vi "Main Tclk.vi"() -> ()   [LabVIEW 2018] (continued)
                n4379 = local write "Faraday Cup before mill"(w3310) -> ()
                n4380 = call <vilib>:"Three Button Dialog.vi"("Allow user to close window? (TRUE)"=FALSE, "Center Button Text (\"No\")"="Manual Re-engage" ("T button name (\"OK\")"), "Left Button Text (\"Yes\")"="Auto Re-engage" ("T button name (\"OK\")"), "message"="Reheat finish and ready to re-engage?") -> ("Which Button?"=w3313:T78)  [unwired: 7 in]
                n4381 = case shown="\"Left Button\"" w3313 {
                  frame "Left Button" {
                    n4382 = stacked-sequence {
                      frame #0 {
                        w3352 = dbl[] [] ("Re-engage Delta X array")
                        w3341 = u8 0 ("Re-engage X shift")
                        w3344 = TRUE ("Auto re-engage")
                        n4383 = local read "X shift from last"() -> (w3346:dbl)
                        n4384 = local read "Y shift from last"() -> (w3350:dbl)
                        n4385 = local read "Reheat from last"() -> (w3347:bool)
                        n4386 = local read "FIB-SEM Angle"() -> (w3355:dbl)
                        n4387 = Get Date/Time In Seconds() -> (seconds since 1Jan1904=w3353:timestamp)
                        "Re-engage time" <- w3353
                        n4388 = local read "Pre-reheat time"() -> (w3356:timestamp)
                        n4389 = Subtract(x=w3353, y=w3356) -> (x-y=w3357:dbl)
                        n4390 = expression code="x/60"(w3357) -> (w3358:dbl)
                        n4391 = expression code="cos(x*pi/180)"(w3355) -> (w3354:dbl)
                        n4392 = Select(t=w3346, s=w3347, f=0.0 ("Re-engage X shift")) -> (s? t:f=w3349:dbl)
                        n4393 = Natural Logarithm(1:w3358) -> (0:w3360:dbl)
                        n4394 = local write "Status message"("Auto re-engaging ..." ("Status message")) -> ()
                        n4395 = shared-variable ".\\Zeiss Library.lvlib\\FIB PID reset"(w3344) -> ()  [unwired: 1 in, 1 out]
                        n4396 = local write "Re-engage X shift (um)"(w3349) -> ()
                        n4397 = Compound Arithmetic op=MULTIPLY(w3354, w3360, 2.5 ("value"), 0.0 ("value")) -> (w3351:dbl)
                        n4398 = Select(t=w3350, s=w3347, f=w3351) -> (s? t:f=w3345:dbl)
                        n4399 = local write "Re-engage Y shift (um)"(w3345) -> ()
                        n4400 = local read "Last milling snapshot"() -> (w3337:path)
                        n4401 = local write "Status Tabs"(T11."Status" ("Status Tabs")) -> ()
                        n4402 = call-poly <vilib>:"Read From XML File.vi"("XML File Path"=w3337) -> ("XML Elements"=w3338:string)  [unwired: 8 in, 2 out]
                        n4403 = local write "Re-engage counts"(w3341) -> ()
                        n4404 = local write "Recovered counts"(w3341) -> ()
                        n4405 = local write "Last re-engage count"(w3341) -> ()
                        n4406 = Unflatten From XML(xml string=w3338, type=T46 {"Timestamp"=timestamp(0 s since 1904-01-01), "Milling Z voltage"=0.0, "FIB slice #"=0, "Pause for reheat"=FALSE, "Last good FI"=0.0, "Focus index"=0.0, "SEM max FOV"=0.0, "Remaining X shift frames"=0, "Remaining Y shift frames"=0} ("output cluster")) -> (value=w3336:T46)  [unwired: 1 in, 1 out]
                        n4407 = local write "Image Tabs"(T37."Logging: Realtime Graphs" ("Image Tabs")) -> ()
                        n4408 = Unbundle By Name(w3336) -> ("Milling Z voltage"=w3335:sgl)
                        n4409 = shared-variable ".\\Zeiss Library.lvlib\\Milling Z Voltage Last"(w3335) -> ()  [unwired: 1 in, 1 out]
                        "Auto re-engage" <- w3344
                        "Re-engage Delta X array" <- w3352
                        "Re-engage Delta Y array" <- w3352
                        "Re-engage Y shift array" <- w3352
                        "Re-engage X shift array" <- w3352
                      }
                      frame #1 {
                        w3364 = TRUE ("Reset WD")
                        w3365 = FALSE ("Reheat")
                        n4410 = local write "Config Tabs"(T24."SEM" ("Config Tabs")) -> ()
                        n4411 = local write "Image Tabs"(T37."Detector A" ("Image Tabs")) -> ()
                        n4412 = local write "Pause for reheat"(w3365) -> ()
                        n4413 = local write "Mill Manual Pause"(w3365) -> ()
                        n4414 = local write "Reheat from last"(w3365) -> ()
                        n4415 = property on="Mill Manual Pause" class="Bool (strict)"("DisabledEnum"=T44."Enabled" ("Disabled")) -> ()  [unwired: 2 in, 2 out]
                        n4416 = local write "3D image paused armed"(w3364) -> ()
                        n4417 = local write "SW error warning armed"(w3364) -> ()
                        n4418 = local write "Temperature warning armed"(w3364) -> ()
                        n4419 = local read "Alert Settings"() -> (→"Prior Alert Settings":T36)
                      }
                    }
                  }
                  frame "Center Button", Default {
                    w3375 = TRUE ("Reset WD")
                    w3377 = FALSE ("Reheat")
                    n4420 = local write "3D image paused armed"(w3375) -> ()
                    n4421 = local write "Reset Focus"(w3375) -> ()
                    n4422 = local write "SW error warning armed"(w3375) -> ()
                    n4423 = shared-variable ".\\Zeiss Library.lvlib\\FIB PID reset"(w3375) -> ()  [unwired: 1 in, 1 out]
                    n4424 = local write "Temperature warning armed"(w3375) -> ()
                    n4425 = local write "Status message"("Manual re-engaging ..." ("Status message")) -> ()
                    n4426 = local write "Config Tabs"(T24."SEM" ("Config Tabs")) -> ()
                    n4427 = local write "Status Tabs"(T11."Status" ("Status Tabs")) -> ()
                    n4428 = local write "Image Tabs"(T37."Logging: Realtime Graphs" ("Image Tabs")) -> ()
                    n4429 = local write "Pause for reheat"(w3377) -> ()
                    n4430 = local write "Mill Manual Pause"(w3377) -> ()
                    n4431 = local write "Reheat from last"(w3377) -> ()
                    n4432 = property on="Mill Manual Pause" class="Bool (strict)"("DisabledEnum"=T44."Enabled" ("Disabled")) -> ()  [unwired: 2 in, 2 out]
                    n4433 = local read "Last milling snapshot"() -> (w3370:path)
                    n4434 = call-poly <vilib>:"Read From XML File.vi"("XML File Path"=w3370) -> ("XML Elements"=w3371:string)  [unwired: 8 in, 2 out]
                    n4435 = Unflatten From XML(xml string=w3371, type=T46 {"Timestamp"=timestamp(0 s since 1904-01-01), "Milling Z voltage"=0.0, "FIB slice #"=0, "Pause for reheat"=FALSE, "Last good FI"=0.0, "Focus index"=0.0, "SEM max FOV"=0.0, "Remaining X shift frames"=0, "Remaining Y shift frames"=0} ("output cluster")) -> (value=w3369:T46)  [unwired: 1 in, 1 out]
                    n4436 = Unbundle By Name(w3369) -> ("Milling Z voltage"=w3368:sgl)
                    n4437 = shared-variable ".\\Zeiss Library.lvlib\\Milling Z Voltage Last"(w3368) -> ()  [unwired: 1 in, 1 out]
                  }
                  frame "Right Button" {
                    n4438 = local write "Pause for reheat"(TRUE ("Reheat request")) -> ()
                  }
                }
              }
              frame True {
                n4439 = local read "Mill Manual Pause"() -> (w3393:bool)
                n4440 = Get Date/Time In Seconds() -> (seconds since 1Jan1904=w3391:timestamp)
                n4441 = local read "3D FIB-SEM Files"() -> (w3383:path)
                n4442 = local read "Re-engage Files"() -> (w3381:path)
                n4443 = local read "Last good FI"() -> (w3390:sgl)
                n4444 = case shown="True" w3393 {
                  frame False {
                    n4445 = stacked-sequence {
                      frame #0 {
                        n4446 = local write "Pause for reheat"(FALSE ("Reheat")) -> ()
                      }
                      frame #1 {
                        n4447 = Two Button Dialog(message="Pause to reheat FIB source?") -> (T button?=w3395:bool)  [unwired: 2 in]
                        n4448 = local write "Pause for reheat"(w3395) -> ()
                        n4449 = case shown="True" w3395 {
                          frame False {
                          }
                          frame True {
                            n4450 = local write "Reheat completed"(FALSE ("Reheat completed")) -> ()
                            n4451 = local write "Status message"("Pausing for FIB reheat ..." ("Status message")) -> ()
                            n4452 = property on="Pause for reheat" class="Bool (strict)"("DisabledEnum"=T44."Disabled and Grayed Out" ("Disabled")) -> ()  [unwired: 2 in, 2 out]
                          }
                        }
                      }
                    }
                  }
                  frame True {
                    n4453 = property on="Mill Manual Pause" class="Bool (strict)"("DisabledEnum"=T44."Disabled and Grayed Out" ("Disabled")) -> ()  [unwired: 2 in, 2 out]
                  }
                }
                n4454 = local read "SEM Scan Parameters"() -> (w3392:T26)
                n4455 = Build Path(base path=w3383, name or relative path="LG low res.png") -> (appended path=w3384:path)
                n4456 = Build Path(base path=w3381, name or relative path="pre.png") -> (appended path=w3385:path)
                n4457 = local write "Pre-reheat time"(w3391) -> ()
                n4458 = Copy(9:TRUE ("overwrite (F)"), 10:w3385, 11:w3384) -> ()  [unwired: 2 in, 3 out]
                n4459 = local write "Pre-reheat FI"(w3390) -> ()
                n4460 = Unbundle By Name(w3392) -> ("X center (um)"=w3389:sgl, "Y center (um)"=w3388:sgl, "Y stig"=w3387:sgl[][])
                n4461 = local write "Pre-reheat X center (um)"(w3389) -> ()
                n4462 = local write "Pre-reheat Y center (um)"(w3388) -> ()
                n4463 = local write "Pre-reheat Y stig"(w3387) -> ()
              }
            }
          }
          event "FIB Imaging": Mouse Down {
            n4464 = event-data() -> ("PlatMods"=w3402:T77)  [unwired: 7 out]
            n4465 = Unbundle By Name(w3402) -> ("Shift"=→"FIB single scan":bool)
          }
          event "FIB Imaging": Value Change {
            n4466 = event-data() -> ("NewVal"=w3403:bool)  [unwired: 5 out]
            n4467 = case shown="True" w3403 {
              selector: w3403 -> [w3404 _]
              frame False {
                n4468 = local write "Unfreeze"(w3404) -> ()
                n4469 = stacked-sequence {
                  frame #0 {
                    n4470 = shared-variable "My Computer\\Zeiss Library.lvlib\\Realtime Imaging stop"(TRUE ("Realtime Imaging stop")) -> ()  [unwired: 1 in, 1 out]
                  }
                  frame #1 {
                    n4471 = disable-structure shown="Disabled" {
                      frame Disabled {
                        n4472 = local read "Machine Type"() -> (w3406:u8)
                        n4473 = case shown="1" w3406 {
                          frame 0, Default {
                          }
                          frame 1 {
                            n4474 = stacked-sequence {
                              frame #0 {
                                n4475 = Wait (ms)(milliseconds to wait=u32 1000) -> ()  [unwired: 1 out]
                              }
                              frame #1 {
                                w3408 = TRUE ("Initialization")
                                n4476 = local read "COM port"() -> (w3414:refnum<visa-resource-name>)
                                n4477 = call "FIB mode.vi"("Initialization"=w3408, "FIB mode"=T10."SEM", "COM port in"=w3414) -> ("COM port out"=w3413:refnum<visa-resource-name>)  [unwired: 7 in, 1 out]
                                n4478 = call "Remcon32 command.vi"("SEM command"="edx 0", "COM port in"=w3413) -> ("COM port out"=w3412:refnum<visa-resource-name>)  [unwired: 6 in, 3 out]
                                n4479 = call "Remcon32 command.vi"("Close session"=w3408, "SEM command"="frez", "COM port in"=w3412) -> ()  [unwired: 5 in, 4 out]
                              }
                            }
                          }
                          frame 2 {
                          }
                        }
                      }
                      frame Enabled {
                      }
                    }
                  }
                  frame #2 {
                    w3416 = T44."Enabled" ("Disabled")
                    n4480 = local write "Status message"("standby" ("Status message")) -> ()
                    n4481 = property on="Pre image" class="Bool (strict)"("DisabledEnum"=w3416) -> ()  [unwired: 2 in, 2 out]
                    n4482 = property on="Post image" class="Bool (strict)"("DisabledEnum"=w3416) -> ()  [unwired: 2 in, 2 out]
                    n4483 = local read "FIB"() -> (w3417:bool)
                    n4484 = property on="Mill Manual Pause" class="Bool (strict)"("DisabledEnum"=w3416) -> ()  [unwired: 2 in, 2 out]
                    n4485 = case shown="False" w3417 {
                      tunnel: w3416 -> [w3418 _]
                      frame False {
                        n4486 = property on="Mill" class="Bool (strict)"("DisabledEnum"=w3418) -> ()  [unwired: 2 in, 2 out]
                      }
                      frame True {
                      }
                    }
                  }
                }
              }
              frame True {
                n4487 = local read "Machine Type"() -> (w3420:u8)
                n4488 = case shown="2" w3420 {
                  tunnel: [TRUE ("true") w3432] -> w3419
                  frame 0, Default {
                  }
                  frame 2 {
                    n4489 = local read "Api"() -> (w3430:refnum<k7>)
                    n4490 = Two Button Dialog(message="Verify if FIB probe is at 50 pA") -> (T button?=w3432:bool)  [unwired: 2 in]
                    n4491 = call "SmartSEM Remote API set string.vi"("vValue"="FIB Imaging Probe", "lpszParam"="DP_FIB_IMAGE_PROBE", "ActiveX Container"=w3430) -> ()  [unwired: 7 in, 2 out]
                  }
                }
                "Unfreeze" <- w3419
                n4492 = case shown="True" w3419 {
                  frame False {
                  }
                  frame True {
                    n4493 = stacked-sequence {
                      frame #0 {
                        n4494 = local read "Spot"() -> (w3421:bool)
                        n4495 = case shown="True" w3421 {
                          frame False {
                          }
                          frame True {
                            n4496 = local write "Spot"(FALSE ("Spot")) -> ()
                            n4497 = Wait (ms)(milliseconds to wait=u32 200) -> ()  [unwired: 1 out]
                          }
                        }
                      }
                      frame #1 {
                        w3426 = T44."Disabled and Grayed Out" ("Disabled")
                        n4498 = local write "Status message"("FIB Imaging" ("Status message")) -> ()
                        n4499 = local write "Image Tabs"(T37."FIB" ("Image Tabs")) -> ()
                        n4500 = local write "Status Tabs"(T11."FIB" ("Status Tabs")) -> ()
                        n4501 = property on="Pre image" class="Bool (strict)"("DisabledEnum"=w3426) -> ()  [unwired: 2 in, 2 out]
                        n4502 = property on="Post image" class="Bool (strict)"("DisabledEnum"=w3426) -> ()  [unwired: 2 in, 2 out]
                        n4503 = property on="Mill" class="Bool (strict)"("DisabledEnum"=w3426) -> ()  [unwired: 2 in, 2 out]
                        n4504 = property on="Mill Manual Pause" class="Bool (strict)"("DisabledEnum"=w3426) -> ()  [unwired: 2 in, 2 out]
                      }
                    }
                  }
                }
                n4505 = local write "FIB Imaging"(w3419) -> ()
              }
            }
          }
          event "Update": Value Change {
            n4506 = event-data() -> ("NewVal"=w3434:bool)  [unwired: 5 out]
            n4507 = case shown="True" w3434 {
              frame False {
              }
              frame True {
                n4508 = stacked-sequence {
                  frame #0 {
                    n4509 = local write "Unfreeze"(FALSE ("FIB beam blank")) -> ()
                    n4510 = shared-variable "My Computer\\Zeiss Library.lvlib\\Realtime Imaging stop"(TRUE ("Realtime Imaging stop")) -> ()  [unwired: 1 in, 1 out]
                  }
                  frame #1 {
                    n4511 = Wait (ms)(milliseconds to wait=u32 1000) -> ()  [unwired: 1 out]
                  }
                  frame #2 {
                    n4512 = local write "Unfreeze"(TRUE ("Realtime Imaging stop")) -> ()
                  }
                }
              }
            }
          }
          event "Reset": Value Change {
            n4513 = event-data() -> ("NewVal"=w3439:bool)  [unwired: 5 out]
            n4514 = case shown="True" w3439 {
              frame False {
              }
              frame True {
                n4515 = stacked-sequence {
                  frame #0 {
                    n4516 = local read "SEM HW Config"() -> (w3461:T9)
                    n4517 = local read "FIB HW Config"() -> (w3457:T23)
                    n4518 = Unbundle By Name(w3461) -> ("SEM X coil"=w3449:refnum<k15>, "SEM Y coil"=w3448:refnum<k15>, "Detectors A&B"=w3442:refnum<k15>)
                    n4519 = Unbundle By Name(w3457) -> ("FIB X coil"=w3456:tag)
                    n4520 = Type Cast(x=w3456) -> (*(type *) &x=w3458:string)  [unwired: 1 in]
                    n4521 = Match Pattern(string=w3458, regular expression="/") -> (before substring=w3460:string)  [unwired: 1 in, 3 out]
                    n4522 = call <instrlib>:"niFgen Initialize.vi"("Resource Name"=w3449) -> ("error out"=w3452:errorcluster, "Instrument Handle Out"=w3451:refnum<k15>)  [unwired: 9 in]
                    n4523 = call <instrlib>:"niFgen Initialize.vi"("Resource Name"=w3448) -> ("error out"=w3446:errorcluster, "Instrument Handle Out"=w3447:refnum<k15>)  [unwired: 9 in]
                    n4524 = call <instrlib>:"niScope Initialize.vi"("resource name"=w3442) -> ("instrument handle"=w3444:refnum<k15>, "error out"=w3443:errorcluster)  [unwired: 13 in]
                    n4525 = call <instrlib>:"niFgen Reset Device.vi"("error in (no error)"=w3452, "Instrument Handle"=w3451) -> ("error out"=w3450:errorcluster, "Instrument Handle Out"=w3454:refnum<k15>)  [unwired: 8 in]
                    n4526 = call <instrlib>:"niFgen Reset Device.vi"("error in (no error)"=w3446, "Instrument Handle"=w3447) -> ("error out"=w3445:errorcluster, "Instrument Handle Out"=w3453:refnum<k15>)  [unwired: 8 in]
                    n4527 = call <instrlib>:"niScope Reset Device.vi"("instrument handle"=w3444, "error in"=w3443) -> ("instrument handle out"=w3441:refnum<k15>, "error out"=w3440:errorcluster)  [unwired: 12 in]
                    n4528 = call <vilib>:"DAQmx Reset Device.vi"("device in"=w3460) -> ()  [unwired: 14 in, 1 out]
                    n4529 = call <instrlib>:"niFgen Self-Test.vi"("error in (no error)"=w3450, "Instrument Handle"=w3454) -> ()  [unwired: 6 in, 4 out]
                    n4530 = call <instrlib>:"niFgen Self-Test.vi"("error in (no error)"=w3445, "Instrument Handle"=w3453) -> ()  [unwired: 6 in, 4 out]
                    n4531 = call <instrlib>:"niScope Self Test.vi"("instrument handle"=w3441, "error in"=w3440) -> ()  [unwired: 10 in, 4 out]
                    n4532 = shared-variable ".\\Zeiss Library.lvlib\\Force tclk init"(TRUE ("Force tclk init")) -> ()  [unwired: 1 in, 1 out]
                  }
                  frame #1 {
                    n4533 = local read "FIB HW Config"() -> (w3472:T23)
                    n4534 = local read "Hardware Configuration"() -> (w3469:T25)
                    n4535 = Unbundle By Name(w3472) -> ("Beam blank"=w3473:tag)
                    n4536 = local read "Api"() -> (w3470:refnum<k7>)
                    n4537 = local read "Damping"() -> (w3462:bool)
                    n4538 = Unbundle By Name(w3469) -> ("Shutter Drive"=w3464:tag)
                    n4539 = call "FIB beam blank.vi"("ActiveX Container"=w3470, "Beam blanked"=TRUE ("Ext on"), "lines"=w3473) -> ()  [unwired: 2 in, 1 out]
                    n4540 = call "Shutter Swing V3.vi"("Shutter Drive"=w3464, "Damping"=w3462, "Shutter close"=FALSE) -> ("Shutter close fdbk"=w3465:bool, "Fail #"=w3467:u8, "SEM shutter status"=w3468:string)  [unwired: 2 in, 4 out]
                    n4541 = Greater Than 0?(x=w3467) -> (x > 0?=w3466:bool)
                    n4542 = local write "SEM shutter status"(w3468) -> ()
                    n4543 = local write "Fail #"(w3467) -> ()
                    n4544 = local write "SEM shutter failed active"(w3466) -> ()
                    n4545 = local write "SEM Shutter"(w3465) -> ()
                  }
                  frame #2 {
                    n4546 = local read "SEM HW Config"() -> (w3478:T9)
                    n4547 = Unbundle By Name(w3478) -> ("Detector FIB-NI auto switch"=w3479:tag)
                    n4548 = call-poly <vilib>:"DAQmx Create Virtual Channel.vi"("lines"=w3479) -> ("task out"=w3476:refnum<k21>, "error out"=w3477:errorcluster)  [unwired: 4 in, 9 out]
                    n4549 = call-poly <vilib>:"DAQmx Write.vi"("task/channels in"=w3476, "data"=FALSE, "error in"=w3477) -> ("task out"=w3474:refnum<k21>, "error out"=w3475:errorcluster)  [unwired: 1 in, 10 out]
                    n4550 = call <vilib>:"DAQmx Clear Task.vi"("task in"=w3474, "error in"=w3475) -> ()  [unwired: 14 out]
                  }
                  frame #3 {
                    w3481 = sgl[] [] ("SEM Specimen I high limit array")
                    n4551 = local read "FIB HW Config"() -> (w3485:T23)
                    n4552 = local write "SEM Specimen I low limit array"(w3481) -> ()
                    n4553 = local write "SEM Specimen I array"(w3481) -> ()
                    n4554 = local write "SEM Specimen I high limit array"(w3481) -> ()
                    n4555 = local write "Specimen I array"(w3481) -> ()
                    n4556 = local write "Specimen I high limit array"(w3481) -> ()
                    n4557 = local write "Specimen I low limit array"(w3481) -> ()
                    n4558 = local write "Milling I array"(w3481) -> ()
                    n4559 = local write "Milling I high limit array"(w3481) -> ()
                    n4560 = local write "Milling I low limit array"(w3481) -> ()
                    n4561 = Unbundle By Name(w3485) -> ("FIB Ext Scan"=w3484:tag)
                    n4562 = call "FIB ext scan.vi"("Ext on"=FALSE, "FIB Ext Scan"=w3484) -> ()  [unwired: 9 in, 1 out]
                    n4563 = local write "Faraday Cup array"(w3481) -> ()
                    n4564 = local write "Faraday Cup high limit array"(w3481) -> ()
                    n4565 = local write "Faraday Cup low limit array"(w3481) -> ()
                    n4566 = local write "Beam Dump 1 array"(w3481) -> ()
                    n4567 = local write "BD1 high limit array"(w3481) -> ()
                    n4568 = local write "BD1 low limit array"(w3481) -> ()
                    n4569 = local write "Beam Dump 2 array"(w3481) -> ()
                    n4570 = local write "BD2 high limit array"(w3481) -> ()
                    n4571 = local write "BD2 low limit array"(w3481) -> ()
                    n4572 = local write "Log time array"(u32[] [] ("Log time array")) -> ()
                    n4573 = local write "Temp low limit array"(w3481) -> ()
                    n4574 = local write "Temp array"(w3481) -> ()
                    n4575 = local write "Temp high limit array"(w3481) -> ()
                    n4576 = local write "Focus index array"(w3481) -> ()
                    n4577 = local write "FRC array"(w3481) -> ()
                    n4578 = local write "Delta X array"(w3481) -> ()
                    n4579 = local write "Delta Y array"(w3481) -> ()
                    n4580 = local write "Delta Z array"(w3481) -> ()
                    n4581 = local write "Delta X sum array"(w3481) -> ()
                    n4582 = local write "Delta Y sum array"(w3481) -> ()
                    n4583 = local write "Delta image array"(w3481) -> ()
                    n4584 = local write "Milling Z voltage array"(w3481) -> ()
                  }
                  frame #4 {
                    n4585 = local read "Machine Type"() -> (w3486:u8)
                    n4586 = case shown="2" w3486 {
                      frame 0, Default {
                      }
                      frame 1 {
                        w3487 = TRUE ("Initialization")
                        n4587 = local read "COM port"() -> (w3493:refnum<visa-resource-name>)
                        n4588 = call "FIB mode.vi"("Initialization"=w3487, "FIB mode"=T10."SEM", "COM port in"=w3493) -> ("COM port out"=w3492:refnum<visa-resource-name>)  [unwired: 7 in, 1 out]
                        n4589 = call "Remcon32 command.vi"("SEM command"="edx 0", "COM port in"=w3492) -> ("COM port out"=w3491:refnum<visa-resource-name>)  [unwired: 6 in, 3 out]
                        n4590 = call "Remcon32 command.vi"("Close session"=w3487, "SEM command"="frez", "COM port in"=w3491) -> ()  [unwired: 5 in, 4 out]
                      }
                      frame 2 {
                        n4591 = local read "Api"() -> (w3494:refnum<k7>)
                        n4592 = call "SmartSEM Remote API set float.vi"("vValue"=sgl 0.0, "lpszParam"="DP_PANEL_DISABLE", "ActiveX Container"=w3494) -> ("reference out"=w3495:refnum<k7>)  [unwired: 7 in, 1 out]
                        n4593 = call "SmartSEM Remote API set float.vi"("vValue"=sgl 0.0, "lpszParam"="DP_JOYSTICK_DISABLE", "ActiveX Container"=w3495) -> ()  [unwired: 7 in, 2 out]
                      }
                    }
                  }
                  frame #5 {
                    n4594 = local write "Reset"(FALSE ("Reset")) -> ()
                  }
                }
              }
            }
          }
          event "Reset Watchdog": Value Change {
            n4595 = event-data() -> ("NewVal"=w3501:bool)  [unwired: 5 out]
            n4596 = case shown="True" w3501 {
              frame False {
              }
              frame True {
                n4597 = local read "WatchDog Mode"() -> (w3502:u16)
                n4598 = flat-sequence {
                  tunnel: w3502 -> [w3503]
                  tunnel: w3502 -> [w3506]
                  frame #0 {
                    n4599 = call "FM Gen Pulse for FIB-SEM.vi"("WatchDog Mode"=w3503, "State Value"=i16 0) -> ()  [unwired: 7 in, 3 out]
                  }
                  frame #1 {
                    n4600 = Wait (ms)(milliseconds to wait=u32 2) -> ()  [unwired: 1 out]
                  }
                  frame #2 {
                    n4601 = call "FM Gen Pulse for FIB-SEM.vi"("WatchDog Mode"=w3506, "State Value"=i16 1) -> ()  [unwired: 7 in, 3 out]
                  }
                  frame #3 {
                    n4602 = Wait (ms)(milliseconds to wait=u32 250) -> ()  [unwired: 1 out]
                  }
                }
              }
            }
          }
          event "Off": Value Change {
            n4603 = event-data() -> ("NewVal"=w3509:bool)  [unwired: 6 out]
            n4604 = case shown="True" w3509 {
              tunnel: [FALSE ("T button?") w3512] -> w3510
              frame False {
              }
              frame True {
                n4605 = local read "FIB"() -> (w3513:bool)
                n4606 = Two Button Dialog(message="Stop Program?") -> (T button?=w3514:bool)  [unwired: 2 in]
                n4607 = case shown="True" w3513 {
                  tunnel: w3514 -> [w3516 w3517]
                  tunnel: [w3516 w3517] -> w3512
                  frame False {
                    n4608 = shared-variable "My Computer\\Zeiss Library.lvlib\\Stop"(w3516) -> ()  [unwired: 1 in, 1 out]
                    n4609 = shared-variable "My Computer\\Zeiss Library.lvlib\\Milling Stop"(w3516) -> ()  [unwired: 1 in, 1 out]
                    n4610 = shared-variable "My Computer\\Zeiss Library.lvlib\\Realtime Imaging stop"(w3516) -> ()  [unwired: 1 in, 1 out]
                    n4611 = local write "Stop"(w3516) -> ()
                    n4612 = local write "Off"(w3516) -> ()
                  }
                  frame True {
                    n4613 = shared-variable "My Computer\\Zeiss Library.lvlib\\Stop"(w3517) -> ()  [unwired: 1 in, 1 out]
                    n4614 = shared-variable "My Computer\\Zeiss Library.lvlib\\Milling Stop"(w3517) -> ()  [unwired: 1 in, 1 out]
                    n4615 = shared-variable "My Computer\\Zeiss Library.lvlib\\Realtime Imaging stop"(w3517) -> ()  [unwired: 1 in, 1 out]
                    n4616 = local write "Stop"(w3517) -> ()
                    n4617 = local write "Off"(w3517) -> ()
                  }
                }
              }
            }
          }
          event "SEM Scan Parameters": Value Change {
            w3519 = sgl[] [] ("Delta X array for stop limit")
            n4618 = event-data() -> ()  [unwired: 6 out]
            n4619 = local write "SW error warning armed"(FALSE ("SW error warning armed")) -> ()
            n4620 = local write "Cycle time array"(u32[] [] ("Cycle time array")) -> ()
            n4621 = local write "Cycle time est offset array"(i16[] [] ("Cycle time array")) -> ()
            n4622 = local write "Continued fine milling frames"(0 ("Continued fine milling frames")) -> ()
            n4623 = local write "FI array for stop limit"(w3519) -> ()
            n4624 = local write "Delta X array for stop limit"(w3519) -> ()
            n4625 = local write "Delta Y array for stop limit"(w3519) -> ()
          }
          event "SEM Scan Parameters.X tiles": Value Change {
            n4626 = event-data() -> ("OldVal"=w3527:u8, "NewVal"=w3526:u8)  [unwired: 5 out]
            n4627 = In Range and Coerce(upper limit=u8 255, x=w3526, lower limit=u8 1) -> (coerced(x)=w3525:u8)  [unwired: 1 out]
            n4628 = call <vilib>:"Three Button Dialog.vi"("Center Button Text (\"No\")"="Manual" ("Center Button Text (\"No\")"), "Left Button Text (\"Yes\")"="Auto" ("message"), "message"="Modify WD, Stig, and Aperture Align?") -> ("Which Button?"=w3530:T78)  [unwired: 8 in]
            n4629 = case shown="\"Left Button\"" w3530 {
              tunnel: w3525 -> [w3532 w3562 _]
              tunnel: w3527 -> [_ _ w3638]
              frame "Left Button" {
                n4630 = local read "SEM Scan Parameters"() -> (w3548:T26)
                n4631 = Unbundle By Name(w3548) -> ("X stig"=w3554:sgl[][], "Y stig"=w3553:sgl[][], "X aln"=w3552:sgl[][], "Y aln"=w3551:sgl[][], "WD (mm)"=w3550:sgl[][], "dY (um)"=w3539:sgl[], "Y tiles"=w3533:u8)
                n4632 = Build Array(w3554, w3553, w3552, w3551, w3550) -> (w3549:sgl[][][])
                n4633 = for {
                  tunnel: w3549 -> [w3557] mode=indexing
                  tunnel: w3532 -> [w3556]
                  tunnel: [w3555] -> w3546 mode=indexing
                  workers-P: _ -> [_]
                  n4634 = for {
                    tunnel: w3557 -> [w3561] mode=indexing
                    tunnel: w3556 -> [w3559]
                    tunnel: [w3558] -> w3555 mode=indexing
                    workers-P: _ -> [_]
                    n4635 = call-poly <vilib>:"Mean.vi"("X"=w3561) -> ("mean"=w3560:dbl)  [unwired: 1 out]
                    n4636 = Initialize Array(w3560, w3559) -> (w3558:dbl[])
                  }
                }
                n4637 = call-poly <vilib>:"Mean.vi"("X"=w3539) -> ("mean"=w3540:dbl)  [unwired: 1 out]
                n4638 = Initialize Array(w3540, w3532) -> (w3538:dbl[])
                n4639 = Initialize Array(u8 1 ("element"), w3533, w3532) -> (w3534:u8[][])
                n4640 = local read "Focus Index Options"() -> (w3536:T28)
                n4641 = Index Array(array=w3546) -> (element #1=w3545:dbl[][], element #2=w3544:dbl[][], element #3=w3543:dbl[][], element #4=w3542:dbl[][], element #5=w3541:dbl[][])  [unwired: 15 in]
                n4642 = Bundle By Name(cluster=w3536, "X Grids"=w3534, "Y Grids"=w3534, "Primary X index"=w3534, "Primary Y index"=w3534) -> (w3535:T28)
                n4643 = Bundle By Name(cluster=w3548, "X stig"=w3545, "Y stig"=w3544, "X aln"=w3543, "Y aln"=w3542, "WD (mm)"=w3541, "dY (um)"=w3538, "X tiles"=w3532) -> (w3547:T26)
                n4644 = local write "SEM Scan Parameters"(w3547) -> ()
                n4645 = local write "Focus Index Options"(w3535) -> ()
              }
              frame "Center Button" {
                n4646 = stacked-sequence {
                  tunnel: w3562 -> [w3563 w3580 w3591 w3603 w3615 w3628]
                  frame #0 {
                    n4647 = local read "SEM Scan Parameters"() -> (w3576:T26)
                    n4648 = Unbundle By Name(w3576) -> ("WD (mm)"=w3578:sgl[][], "Y tiles"=w3564:u8)
                    n4649 = call "2D array edit.vi"("Data Entry Limits:Increment"=0.001, "Display Format:Precision"=u8 4, "Rows"=w3564, "Columns"=w3563, "Caption.Text"="WD (mm)", "Input array"=w3578) -> ("Output array"=w3574:sgl[][])  [unwired: 5 in]
                    n4650 = Array Size(array=w3574) -> (size(s)=w3573:i32[])
                    n4651 = Initialize Array(u8 1 ("element"), w3564, w3563) -> (w3565:u8[][])
                    n4652 = local read "Focus Index Options"() -> (w3567:T28)
                    n4653 = Index Array(array=w3573) -> (element #1=w3572:i32, element #2=w3571:i32)  [unwired: 2 in]
                    n4654 = Bundle By Name(cluster=w3567, "X Grids"=w3565, "Y Grids"=w3565, "Primary X index"=w3565, "Primary Y index"=w3565) -> (w3566:T28)
                    n4655 = Bundle By Name(cluster=w3576, "WD (mm)"=w3574, "X tiles"=w3571, "Y tiles"=w3572) -> (w3575:T26)
                    n4656 = local write "SEM Scan Parameters"(w3575) -> ()
                    n4657 = local write "Focus Index Options"(w3566) -> ()
                  }
                  frame #1 {
                    n4658 = local read "SEM Scan Parameters"() -> (w3588:T26)
                    n4659 = Unbundle By Name(w3588) -> ("X stig"=w3590:sgl[][], "Y tiles"=w3579:u8)
                    n4660 = call "2D array edit.vi"("Data Entry Limits:Increment"=0.1, "Display Format:Precision"=u8 2, "Rows"=w3579, "Columns"=w3580, "Caption.Text"="X stig (%)", "Input array"=w3590) -> ("Output array"=w3585:sgl[][])  [unwired: 5 in]
                    n4661 = Array Size(array=w3585) -> (size(s)=w3586:i32[])
                    n4662 = Index Array(array=w3586) -> (element #1=w3584:i32, element #2=w3583:i32)  [unwired: 2 in]
                    n4663 = Bundle By Name(cluster=w3588, "X stig"=w3585, "X tiles"=w3583, "Y tiles"=w3584) -> (w3587:T26)
                    n4664 = local write "SEM Scan Parameters"(w3587) -> ()
                  }
                  frame #2 {
                    n4665 = local read "SEM Scan Parameters"() -> (w3600:T26)
                    n4666 = Unbundle By Name(w3600) -> ("Y stig"=w3602:sgl[][], "Y tiles"=w3598:u8)
                    n4667 = call "2D array edit.vi"("Data Entry Limits:Increment"=0.1, "Display Format:Precision"=u8 2, "Rows"=w3598, "Columns"=w3591, "Caption.Text"="Y stig (%)", "Input array"=w3602) -> ("Output array"=w3596:sgl[][])  [unwired: 5 in]
                    n4668 = Array Size(array=w3596) -> (size(s)=w3597:i32[])
                    n4669 = Index Array(array=w3597) -> (element #1=w3595:i32, element #2=w3594:i32)  [unwired: 2 in]
                    n4670 = Bundle By Name(cluster=w3600, "Y stig"=w3596, "X tiles"=w3594, "Y tiles"=w3595) -> (w3599:T26)
                    n4671 = local write "SEM Scan Parameters"(w3599) -> ()
                  }
                  frame #3 {
                    n4672 = local read "SEM Scan Parameters"() -> (w3612:T26)
                    n4673 = Unbundle By Name(w3612) -> ("X aln"=w3614:sgl[][], "Y tiles"=w3610:u8)
                    n4674 = call "2D array edit.vi"("Data Entry Limits:Increment"=0.1, "Display Format:Precision"=u8 2, "Rows"=w3610, "Columns"=w3603, "Caption.Text"="X aln (%)", "Input array"=w3614) -> ("Output array"=w3608:sgl[][])  [unwired: 5 in]
                    n4675 = Array Size(array=w3608) -> (size(s)=w3609:i32[])
                    n4676 = Index Array(array=w3609) -> (element #1=w3607:i32, element #2=w3606:i32)  [unwired: 2 in]
                    n4677 = Bundle By Name(cluster=w3612, "X aln"=w3608, "X tiles"=w3606, "Y tiles"=w3607) -> (w3611:T26)
                    n4678 = local write "SEM Scan Parameters"(w3611) -> ()
                  }
                  frame #4 {
                    n4679 = local read "SEM Scan Parameters"() -> (w3624:T26)
                    n4680 = Unbundle By Name(w3624) -> ("Y aln"=w3626:sgl[][], "Y tiles"=w3622:u8)
                    n4681 = call "2D array edit.vi"("Data Entry Limits:Increment"=0.1, "Display Format:Precision"=u8 2, "Rows"=w3622, "Columns"=w3615, "Caption.Text"="Y aln (%)", "Input array"=w3626) -> ("Output array"=w3620:sgl[][])  [unwired: 5 in]
                    n4682 = Array Size(array=w3620) -> (size(s)=w3621:i32[])
                    n4683 = Index Array(array=w3621) -> (element #1=w3619:i32, element #2=w3618:i32)  [unwired: 2 in]
                    n4684 = Bundle By Name(cluster=w3624, "Y aln"=w3620, "X tiles"=w3618, "Y tiles"=w3619) -> (w3623:T26)
                    n4685 = local write "SEM Scan Parameters"(w3623) -> ()
                  }
                  frame #5 {
                    w3631 = u8 1 ("Rows")
                    n4686 = local read "SEM Scan Parameters"() -> (w3636:T26)
                    n4687 = Unbundle By Name(w3636) -> ("dY (um)"=w3632:sgl[])
                    n4688 = Reshape Array(w3632, w3631, w3628) -> (w3630:sgl[][])
                    n4689 = call "2D array edit.vi"("Data Entry Limits:Increment"=0.1, "Display Format:Precision"=u8 2, "Rows"=w3631, "Columns"=w3628, "Caption.Text"="dY (um)", "Input array"=w3630) -> ("Output array"=w3629:sgl[][])  [unwired: 5 in]
                    n4690 = Reshape Array(w3629, w3628) -> (w3627:sgl[])
                    n4691 = Bundle By Name(cluster=w3636, "dY (um)"=w3627, "X tiles"=w3628) -> (w3635:T26)
                    n4692 = local write "SEM Scan Parameters"(w3635) -> ()
                  }
                }
              }
              frame "Right Button", Default {
                n4693 = local read "SEM Scan Parameters"() -> (w3639:T26)
                n4694 = Bundle By Name(cluster=w3639, "X tiles"=w3638) -> (w3640:T26)
                n4695 = local write "SEM Scan Parameters"(w3640) -> ()
              }
            }
          }
          event "SEM Scan Parameters.Y tiles": Value Change {
            n4696 = event-data() -> ("OldVal"=w3645:u8, "NewVal"=w3644:u8)  [unwired: 5 out]
            n4697 = In Range and Coerce(upper limit=u8 255, x=w3644, lower limit=u8 1) -> (coerced(x)=w3643:u8)  [unwired: 1 out]
            n4698 = call <vilib>:"Three Button Dialog.vi"("Center Button Text (\"No\")"="Manual" ("Center Button Text (\"No\")"), "Left Button Text (\"Yes\")"="Auto" ("message"), "message"="Modify WD, Stig, and Aperture Align?") -> ("Which Button?"=w3646:T78)  [unwired: 8 in]
            n4699 = case shown="\"Left Button\"" w3646 {
              tunnel: w3643 -> [w3651 w3682 _]
              tunnel: w3645 -> [_ _ w3758]
              frame "Left Button" {
                n4700 = local read "SEM Scan Parameters"() -> (w3666:T26)
                n4701 = Unbundle By Name(w3666) -> ("X stig"=w3672:sgl[][], "Y stig"=w3671:sgl[][], "X aln"=w3670:sgl[][], "Y aln"=w3669:sgl[][], "WD (mm)"=w3668:sgl[][], "dX (um)"=w3657:sgl[], "X tiles"=w3650:u8)
                n4702 = Build Array(w3672, w3671, w3670, w3669, w3668) -> (w3667:sgl[][][])
                n4703 = for {
                  tunnel: w3667 -> [w3676] mode=indexing
                  tunnel: w3651 -> [w3677]
                  tunnel: [w3673] -> w3664 mode=indexing
                  workers-P: _ -> [_]
                  n4704 = Transpose 2D Array(2D array=w3676) -> (transposed array=w3675:sgl[][])
                  n4705 = for {
                    tunnel: w3677 -> [w3680]
                    tunnel: [w3679] -> w3674 mode=indexing
                    workers-P: _ -> [_]
                    tunnel: w3675 -> [w3678] mode=indexing
                    n4706 = call-poly <vilib>:"Mean.vi"("X"=w3678) -> ("mean"=w3681:dbl)  [unwired: 1 out]
                    n4707 = Initialize Array(w3681, w3680) -> (w3679:dbl[])
                  }
                  n4708 = Transpose 2D Array(2D array=w3674) -> (transposed array=w3673:dbl[][])
                }
                n4709 = call-poly <vilib>:"Mean.vi"("X"=w3657) -> ("mean"=w3658:dbl)  [unwired: 1 out]
                n4710 = Initialize Array(w3658, w3651) -> (w3656:dbl[])
                n4711 = Index Array(array=w3664) -> (element #1=w3663:dbl[][], element #2=w3662:dbl[][], element #3=w3661:dbl[][], element #4=w3660:dbl[][], element #5=w3659:dbl[][])  [unwired: 15 in]
                n4712 = Initialize Array(u8 1 ("element"), w3651, w3650) -> (w3652:u8[][])
                n4713 = local read "Focus Index Options"() -> (w3654:T28)
                n4714 = Bundle By Name(cluster=w3654, "X Grids"=w3652, "Y Grids"=w3652, "Primary X index"=w3652, "Primary Y index"=w3652) -> (w3653:T28)
                n4715 = Bundle By Name(cluster=w3666, "X stig"=w3663, "Y stig"=w3662, "X aln"=w3661, "Y aln"=w3660, "WD (mm)"=w3659, "dX (um)"=w3656, "Y tiles"=w3651) -> (w3665:T26)
                n4716 = local write "SEM Scan Parameters"(w3665) -> ()
                n4717 = local write "Focus Index Options"(w3653) -> ()
              }
              frame "Center Button" {
                n4718 = stacked-sequence {
                  tunnel: w3682 -> [w3683 w3699 w3711 w3723 w3735 w3748]
                  frame #0 {
                    n4719 = local read "SEM Scan Parameters"() -> (w3696:T26)
                    n4720 = Unbundle By Name(w3696) -> ("WD (mm)"=w3698:sgl[][], "X tiles"=w3684:u8)
                    n4721 = call "2D array edit.vi"("Data Entry Limits:Increment"=0.001, "Display Format:Precision"=u8 4, "Rows"=w3683, "Columns"=w3684, "Caption.Text"="WD (mm)", "Input array"=w3698) -> ("Output array"=w3694:sgl[][])  [unwired: 5 in]
                    n4722 = Array Size(array=w3694) -> (size(s)=w3693:i32[])
                    n4723 = Initialize Array(u8 1 ("element"), w3683, w3684) -> (w3685:u8[][])
                    n4724 = local read "Focus Index Options"() -> (w3687:T28)
                    n4725 = Index Array(array=w3693) -> (element #1=w3692:i32, element #2=w3691:i32)  [unwired: 2 in]
                    n4726 = Bundle By Name(cluster=w3687, "X Grids"=w3685, "Y Grids"=w3685, "Primary X index"=w3685, "Primary Y index"=w3685) -> (w3686:T28)
                    n4727 = Bundle By Name(cluster=w3696, "WD (mm)"=w3694, "X tiles"=w3691, "Y tiles"=w3692) -> (w3695:T26)
                    n4728 = local write "SEM Scan Parameters"(w3695) -> ()
                    n4729 = local write "Focus Index Options"(w3686) -> ()
                  }
                  frame #1 {
                    n4730 = local read "SEM Scan Parameters"() -> (w3708:T26)
                    n4731 = Unbundle By Name(w3708) -> ("X stig"=w3710:sgl[][], "X tiles"=w3700:u8)
                    n4732 = call "2D array edit.vi"("Data Entry Limits:Increment"=0.1, "Display Format:Precision"=u8 2, "Rows"=w3699, "Columns"=w3700, "Caption.Text"="X stig (%)", "Input array"=w3710) -> ("Output array"=w3705:sgl[][])  [unwired: 5 in]
                    n4733 = Array Size(array=w3705) -> (size(s)=w3706:i32[])
                    n4734 = Index Array(array=w3706) -> (element #1=w3704:i32, element #2=w3703:i32)  [unwired: 2 in]
                    n4735 = Bundle By Name(cluster=w3708, "X stig"=w3705, "X tiles"=w3703, "Y tiles"=w3704) -> (w3707:T26)
                    n4736 = local write "SEM Scan Parameters"(w3707) -> ()
                  }
                  frame #2 {
                    n4737 = local read "SEM Scan Parameters"() -> (w3720:T26)
                    n4738 = Unbundle By Name(w3720) -> ("Y stig"=w3722:sgl[][], "X tiles"=w3712:u8)
                    n4739 = call "2D array edit.vi"("Data Entry Limits:Increment"=0.1, "Display Format:Precision"=u8 2, "Rows"=w3711, "Columns"=w3712, "Caption.Text"="Y stig (%)", "Input array"=w3722) -> ("Output array"=w3717:sgl[][])  [unwired: 5 in]
                    n4740 = Array Size(array=w3717) -> (size(s)=w3718:i32[])
                    n4741 = Index Array(array=w3718) -> (element #1=w3716:i32, element #2=w3715:i32)  [unwired: 2 in]
                    n4742 = Bundle By Name(cluster=w3720, "Y stig"=w3717, "X tiles"=w3715, "Y tiles"=w3716) -> (w3719:T26)
                    n4743 = local write "SEM Scan Parameters"(w3719) -> ()
                  }
                  frame #3 {
                    n4744 = local read "SEM Scan Parameters"() -> (w3732:T26)
                    n4745 = Unbundle By Name(w3732) -> ("X aln"=w3734:sgl[][], "X tiles"=w3724:u8)
                    n4746 = call "2D array edit.vi"("Data Entry Limits:Increment"=0.1, "Display Format:Precision"=u8 2, "Rows"=w3723, "Columns"=w3724, "Caption.Text"="X aln (%)", "Input array"=w3734) -> ("Output array"=w3729:sgl[][])  [unwired: 5 in]
                    n4747 = Array Size(array=w3729) -> (size(s)=w3730:i32[])
                    n4748 = Index Array(array=w3730) -> (element #1=w3728:i32, element #2=w3727:i32)  [unwired: 2 in]
                    n4749 = Bundle By Name(cluster=w3732, "X aln"=w3729, "X tiles"=w3727, "Y tiles"=w3728) -> (w3731:T26)
                    n4750 = local write "SEM Scan Parameters"(w3731) -> ()
                  }
                  frame #4 {
                    n4751 = local read "SEM Scan Parameters"() -> (w3744:T26)
                    n4752 = Unbundle By Name(w3744) -> ("Y aln"=w3746:sgl[][], "X tiles"=w3736:u8)
                    n4753 = call "2D array edit.vi"("Data Entry Limits:Increment"=0.1, "Display Format:Precision"=u8 2, "Rows"=w3735, "Columns"=w3736, "Caption.Text"="Y aln (%)", "Input array"=w3746) -> ("Output array"=w3741:sgl[][])  [unwired: 5 in]
                    n4754 = Array Size(array=w3741) -> (size(s)=w3742:i32[])
                    n4755 = Index Array(array=w3742) -> (element #1=w3740:i32, element #2=w3739:i32)  [unwired: 2 in]
                    n4756 = Bundle By Name(cluster=w3744, "Y aln"=w3741, "X tiles"=w3739, "Y tiles"=w3740) -> (w3743:T26)
                    n4757 = local write "SEM Scan Parameters"(w3743) -> ()
                  }
                  frame #5 {
                    w3747 = u8 1 ("Rows")
                    n4758 = local read "SEM Scan Parameters"() -> (w3756:T26)
                    n4759 = Unbundle By Name(w3756) -> ("dX (um)"=w3752:sgl[])
                    n4760 = Reshape Array(w3752, w3748, w3747) -> (w3751:sgl[][])
                    n4761 = call "2D array edit.vi"("Data Entry Limits:Increment"=0.1, "Display Format:Precision"=u8 2, "Rows"=w3748, "Columns"=w3747, "Caption.Text"="dX (um)", "Input array"=w3751) -> ("Output array"=w3750:sgl[][])  [unwired: 5 in]
                    n4762 = Reshape Array(w3750, w3748) -> (w3749:sgl[])
                    n4763 = Bundle By Name(cluster=w3756, "dX (um)"=w3749, "Y tiles"=w3748) -> (w3755:T26)
                    n4764 = local write "SEM Scan Parameters"(w3755) -> ()
                  }
                }
              }
              frame "Right Button", Default {
                n4765 = local read "SEM Scan Parameters"() -> (w3759:T26)
                n4766 = Bundle By Name(cluster=w3759, "Y tiles"=w3758) -> (w3760:T26)
                n4767 = local write "SEM Scan Parameters"(w3760) -> ()
              }
            }
          }
          event "SEM Scan Parameters.WD (mm)": Mouse Down; "SEM Scan Parameters.WD (mm)": Value Change {
            n4768 = event-data() -> ()  [unwired: 5 out]
            n4769 = local read "SEM Scan Parameters"() -> (w3770:T26)
            n4770 = Unbundle By Name(w3770) -> ("WD (mm)"=w3772:sgl[][], "X tiles"=w3768:u8, "Y tiles"=w3767:u8)
            n4771 = call "2D array edit.vi"("Data Entry Limits:Increment"=0.001, "Display Format:Precision"=u8 4, "Rows"=w3767, "Columns"=w3768, "Caption.Text"="WD (mm)", "Input array"=w3772) -> ("Output array"=w3766:sgl[][])  [unwired: 5 in]
            n4772 = Array Size(array=w3766) -> (size(s)=w3765:i32[])
            n4773 = Index Array(array=w3765) -> (element #1=w3764:i32, element #2=w3763:i32)  [unwired: 2 in]
            n4774 = Bundle By Name(cluster=w3770, "WD (mm)"=w3766, "X tiles"=w3763, "Y tiles"=w3764) -> (w3769:T26)
            n4775 = local write "SEM Scan Parameters"(w3769) -> ()
          }
          event "SEM Scan Parameters.X stig": Mouse Down; "SEM Scan Parameters.X stig": Value Change {
